vi "DAQ.44xx.Get Master and Slave Tasks.vi"(8 "error in (no error)":errorcluster, 10 "AI tasks in":refnum<k21>[](array[refnum]), 11 "AI task":refnum<k21>) -> (0 "error out":errorcluster, 2 "master task":refnum<k21>, 3 "AI task out":refnum<k21>)   [LabVIEW 2019, in "Instrument.DAQ.lvclass"]
uses:
  Instrument.DAQ.lvclass
  <userlib>/_OpenG.lib/array/array.llb/Search 1D Array (U32)__ogtk.vi
  <userlib>/_OpenG.lib/array/array.llb/Index 1D Array Elements (U32)__ogtk.vi
  <resource>/objmgr/daqmx.rc
panel:
  out "x-y":dbl
  out "Slots":u32[](array[numeric])
  out "Chassis":u32[](array[numeric])
  out "Devices":tag[](array[tag])
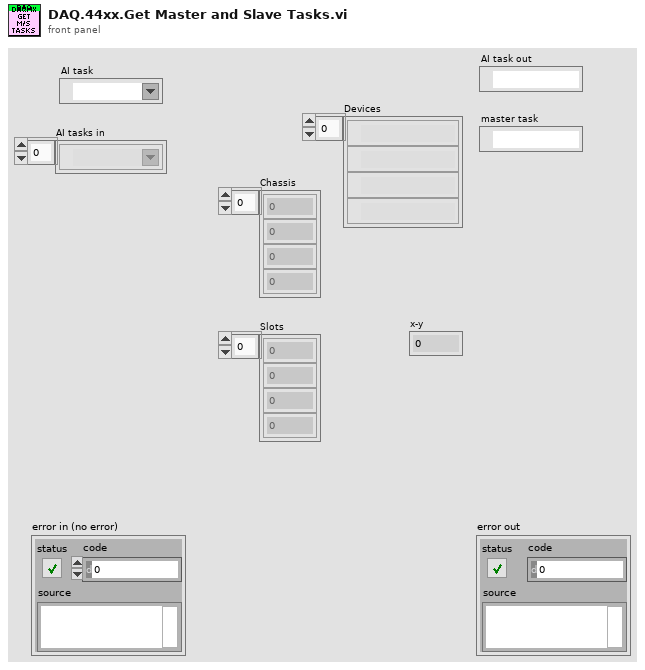
[diagram p1: front panel]
types:
  T1 = typedef "Instrument.DAQ.lvclass/DAQ.Type--enum.ctl" = enum16{"None", "USB-4431", "PXI-446x"}
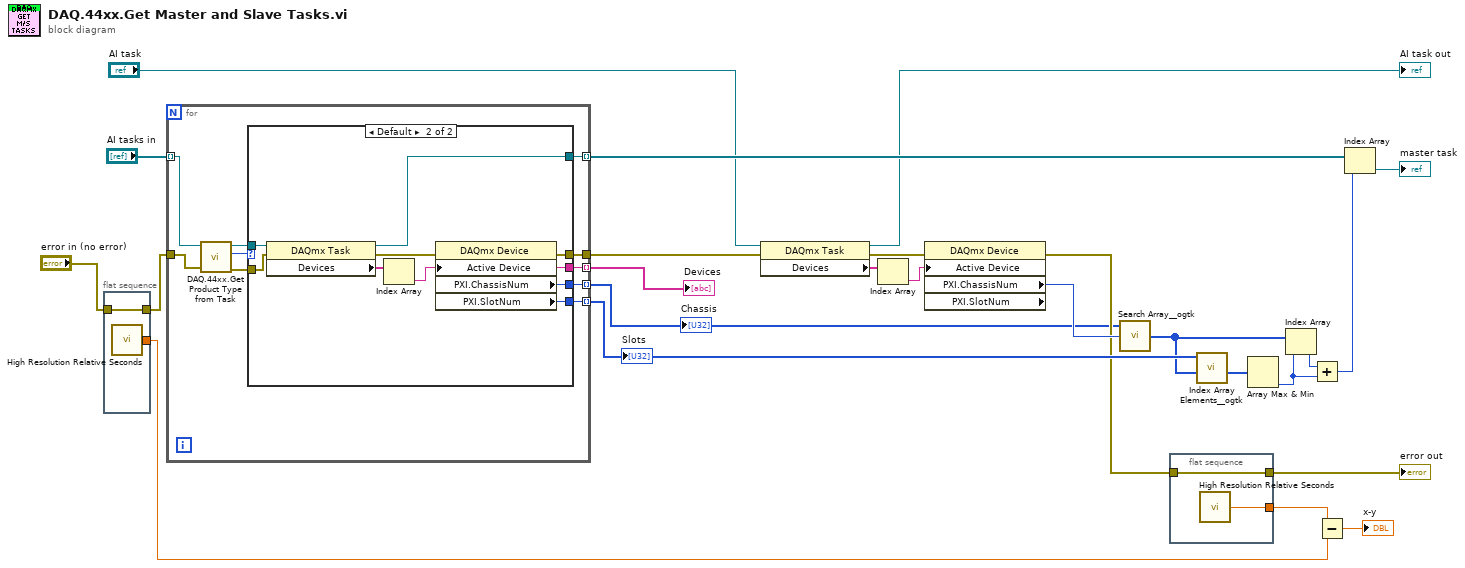
[diagram p0: block diagram]
diagram:
  n1 = flat-sequence {
    tunnel: [w27] -> w14
    tunnel: "error in (no error)" -> [w27]
    tunnel: [w26] -> w9
    frame #0 {
      n2 = call <vilib>:"High Resolution Relative Seconds.vi"() -> ("relative seconds"=w26:dbl)
    }
  }
  n3 = for {
    tunnel: "AI tasks in" -> [w31] mode=indexing
    tunnel: [w33] -> w15 mode=indexing
    tunnel: [w37] -> w1 mode=indexing
    tunnel: [w35] -> w24 mode=indexing
    tunnel: [w36] -> w18 mode=indexing
    tunnel: [w34] -> w20
    tunnel: w14 -> [w29]
    n4 = call "DAQ.44xx.Get Product Type from Task.vi"("error in (no error)"=w29, "Refnum in"=w31) -> ("error out"=w30:errorcluster, "DAQ Type"=w28:T1, "Refnum out"=w32:refnum<k21>)  [unwired: 6 in, 1 out]
    n5 = case shown="Default" w28 {
      tunnel: [_ w46] -> w37
      tunnel: [_ w45] -> w36
      tunnel: [_ w44] -> w35
      tunnel: [w38 w43] -> w34
      tunnel: [w39 w42] -> w33
      tunnel: w32 -> [w39 w41]
      tunnel: w30 -> [w38 w40]
      frame "USB-4431" {
      }
      frame Default {
        n6 = property class="DAQmx Task"(reference=w41, error in=w40) -> (reference out=w42:refnum<k21>, error out=w48:errorcluster, "Devices"=w47:tag[])
        n7 = Index Array(array=w47) -> (element=w44:tag)  [unwired: 1 in]
        n8 = property class="DAQmx Device"(error in=w48, "Active Device"=w44) -> (error out=w43:errorcluster, "PXI.ChassisNum"=w46:u32, "PXI.SlotNum"=w45:u32)  [unwired: 1 in, 1 out]
      }
    }
  }
  "Devices" <- w24
  "Chassis" <- w1
  "Slots" <- w18
  n9 = property class="DAQmx Task"(reference="AI task", error in=w20) -> (reference out=→"AI task out":refnum<k21>, error out=w21:errorcluster, "Devices"=w22:tag[])
  n10 = Index Array(array=w22) -> (element=w23:tag)  [unwired: 1 in]
  n11 = property class="DAQmx Device" props=["Active Device", "PXI.ChassisNum", "PXI.SlotNum"](error in=w21, "Active Device"=w23) -> (error out=w11:errorcluster, "PXI.ChassisNum"=w19:u32)  [unwired: 1 in, 2 out]
  n12 = call-poly <userlib>:"Search Array__ogtk.vi"("Array"=w1, "Element Data"=w19) -> ("Indices of Elements"=w7:i32[])  [unwired: 7 in]
  n13 = flat-sequence {
    tunnel: [w50] -> w12
    tunnel: w11 -> [w50]
    tunnel: [w49] -> w10
    frame #0 {
      n14 = call <vilib>:"High Resolution Relative Seconds.vi"() -> ("relative seconds"=w49:dbl)
    }
  }
  n15 = call-poly <userlib>:"Index Array Elements__ogtk.vi"("indices"=w7, "array"=w18) -> ("elements"=w17:u32[])  [unwired: 9 in]
  n16 = Array Max & Min(array=w17) -> (min index (indices)=w6:i32)  [unwired: 3 out]
  n17 = Index Array(array=w7, index=w6) -> (element=w5:i32)
  n18 = Add(x=w5, y=w6) -> (x+y=w2:i32)
  n19 = Subtract(x=w10, y=w9) -> (x-y=→"x-y":dbl)
  n20 = Index Array(array=w15, index=w2) -> (element=→"master task":refnum<k21>)
  "error out" <- w12
